vi "Object separator.vi"(8 "error in (no error)":errorcluster, 11 "json path in":string="$.home.room.table.lamp") -> (0 "error out":errorcluster, 3 "output array of keys":string[](array[string]))   [LabVIEW 2015]
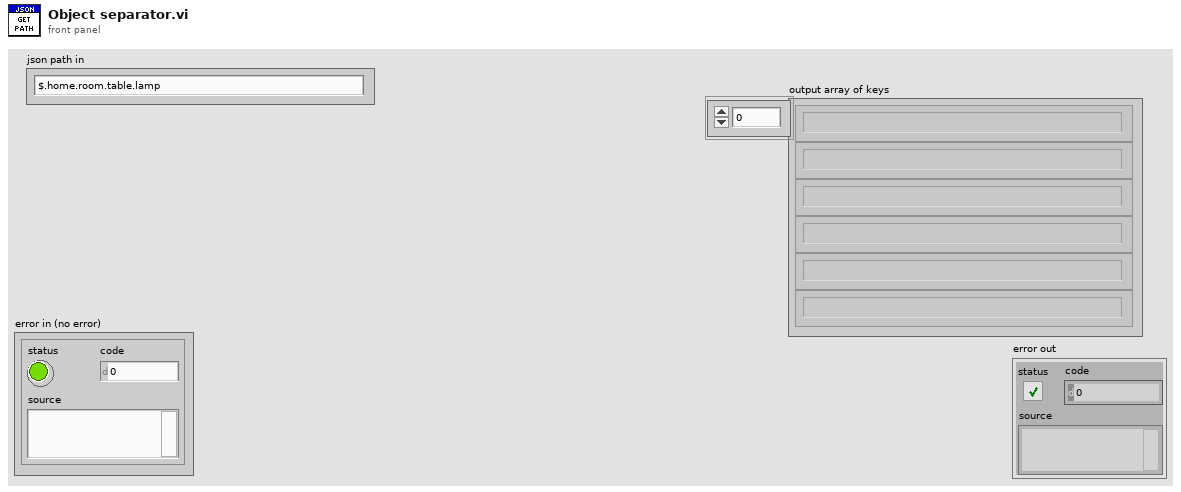
[diagram p1: front panel]
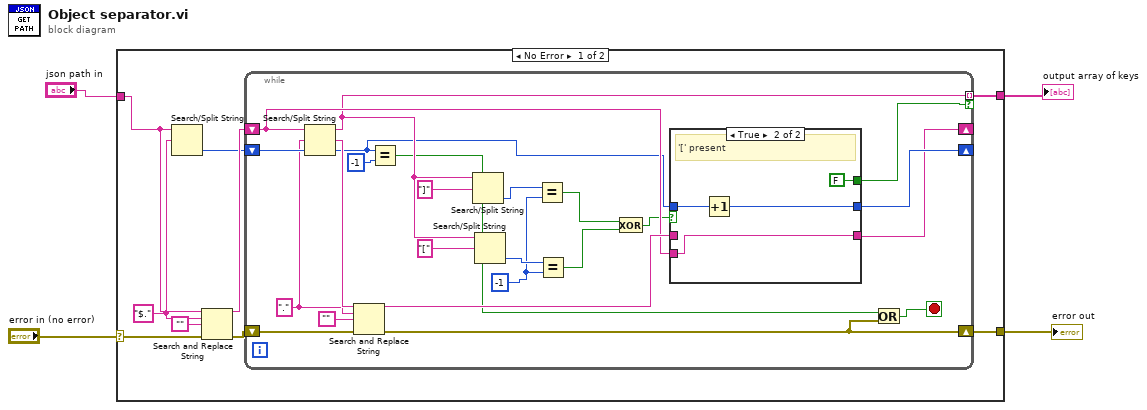
[diagram p0: block diagram]
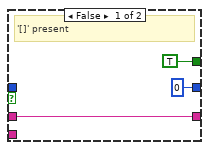
[diagram p2: hidden frame]
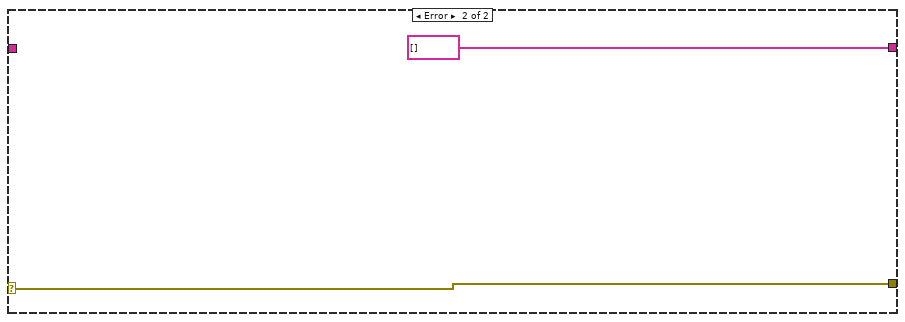
[diagram p3: hidden frame]
diagram:
  n1 = case shown="No Error" "error in (no error)" {
    selector: "error in (no error)" -> [w5 w45]
    tunnel: "json path in" -> [w10 _]
    tunnel: [w7 w45] -> w2
    tunnel: [w8 string[] []] -> w1
    frame No Error {
      w13 = "$." ("search string/char (-)")
      n2 = Search/Split String(string=w10, search string/char (-)=w13) -> (offset of match=w6:i32)  [unwired: 1 in, 2 out]
      n3 = Search and Replace String(input string=w10, search string=w13, replace string="", error in=w5) -> (result string=w11:string, error out=w9:errorcluster)  [unwired: 4 in, 2 out]
      n4 = while {
        shift-right: [w28] -> _
        shift-left: w11 -> [w26]
        tunnel: [w25] -> w8 mode=indexing if=w19
        shift-right: [w14] -> w7
        shift-left: w9 -> [w34]
        shift-right: [w31] -> _
        shift-left: w6 -> [w30]
        stop <- w15 stop-if-true
        w22 = -1 ("y")
        w27 = "." ("search string/char (-)")
        n5 = Search/Split String(string=w26, search string/char (-)=w27, offset (0)=w30) -> (substring before match=w25:string, match + rest of string=w35:string, offset of match=w20:i32)
        n6 = Search and Replace String(input string=w35, search string=w27, replace string="", error in=w34) -> (result string=w29:string, error out=w14:errorcluster)  [unwired: 4 in, 2 out]
        n7 = Equal?(x=w20, y=-1) -> (x = y?=w16:bool)
        n8 = Search/Split String(string=w25, search string/char (-)="]") -> (offset of match=w23:i32)  [unwired: 1 in, 2 out]
        n9 = Search/Split String(string=w25, search string/char (-)="[") -> (offset of match=w32:i32)  [unwired: 1 in, 2 out]
        n10 = Equal?(x=w23, y=w22) -> (x = y?=w18:bool)
        n11 = Equal?(x=w32, y=w22) -> (x = y?=w17:bool)
        n12 = Exclusive Or(1:w17, 2:w18) -> (0:w21:bool)
        n13 = case shown="True" w21 {
          tunnel: w20 -> [_ w43]
          tunnel: [0 w42] -> w31
          tunnel: w29 -> [w39 _]
          tunnel: [w39 w44] -> w28
          tunnel: w26 -> [_ w44]
          tunnel: [TRUE FALSE] -> w19
          frame False {
            # "'[]' present"
          }
          frame True {
            # "'[' present"
            n14 = Increment(x=w43) -> (x+1=w42:i32)
          }
        }
        n15 = Or(x=w16, y=w14) -> (x .or. y?=w15:bool)
      }
    }
    frame Error {
    }
  }
  "output array of keys" <- w1
  "error out" <- w2
